vi "(SubVI)calculate sensitivity vs power.vi"(3 "Convf-cal-array":dbl[](array[numeric]), 4 "Fc-cal-array":dbl[](array[numeric]), 5 "laser power (mW)":dbl) -> (0 "conversion factor (V/um)":dbl, 2 "force constant (pN/nm)":dbl)   [LabVIEW 2014]
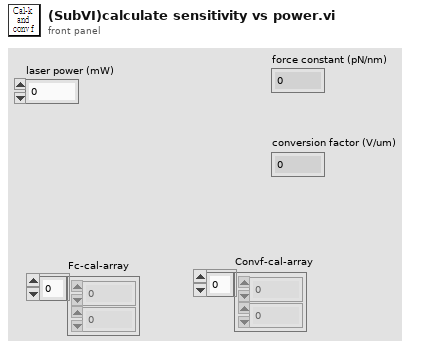
[diagram p1: front panel]
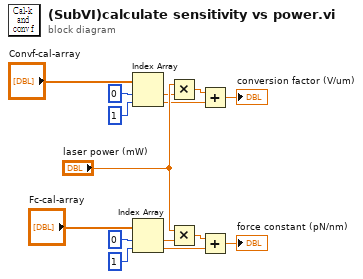
[diagram p0: block diagram]
diagram:
  n1 = Index Array(array="Convf-cal-array", index #1=0 ("index"), index #2=1 ("index")) -> (element #1=w4:dbl, element #2=w3:dbl)
  n2 = Index Array(array="Fc-cal-array", index #1=0 ("index"), index #2=1 ("index")) -> (element #1=w2:dbl, element #2=w1:dbl)
  n3 = Multiply(x="laser power (mW)", y=w4) -> (x*y=w15:dbl)
  n4 = Multiply(x="laser power (mW)", y=w2) -> (x*y=w12:dbl)
  n5 = Add(x=w15, y=w3) -> (x+y=→"conversion factor (V/um)":dbl)
  n6 = Add(x=w12, y=w1) -> (x+y=→"force constant (pN/nm)":dbl)
